vi "[BOOL] to [U8].vi"(1 "[BOOL]":bool[][](array[boolean])) -> (0 "[U8]":u8[][](array[numeric]))   [LabVIEW 2026, in "GoL.lvlib"]
uses:
  GoL.lvlib
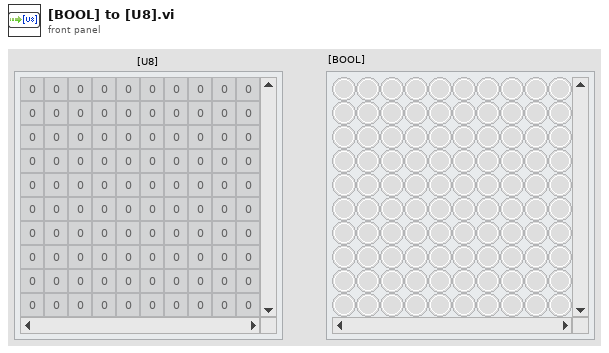
[diagram p1: front panel]
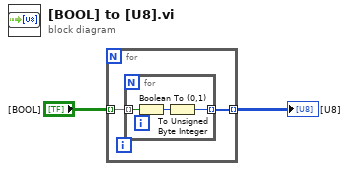
[diagram p0: block diagram]
diagram:
  n1 = for {
    tunnel: "[BOOL]" -> [w4] mode=indexing
    tunnel: [w3] -> w1 mode=indexing
    n2 = for {
      tunnel: w4 -> [w7] mode=indexing
      tunnel: [w5] -> w3 mode=indexing
      n3 = Boolean To (0,1)(Boolean=w7) -> (0, 1=w6:i16)
      n4 = To Unsigned Byte Integer(number=w6) -> (unsigned 8bit integer=w5:u8)
    }
  }
  "[U8]" <- w1
